vi "LinxI2cOpen.vi"(8 "Error In":errorcluster, 10 "I2C Channel":u8, 11 "LINX Resource":T1) -> (0 "Error Out":errorcluster, 3 "LINX Resource":T1)   [LabVIEW 2020, in "LMH-LINX.lvlib" / "Local IO.lvlib"]
uses:
  Local IO.lvlib
  Type Defs/LINX Ref.ctl
  Type Defs/Platform.ctl
  Type Defs/Interface.ctl
  Device/Type Defs/LINX Device Config.ctl
  Device/Type Defs/TCP Config.ctl
  Device/Type Defs/Channels.ctl
  <vilib>/MakerHub/LINX/Resources/liblinxdevice.dll
  LMH-LINX.lvlib
  Device/Device.lvlib
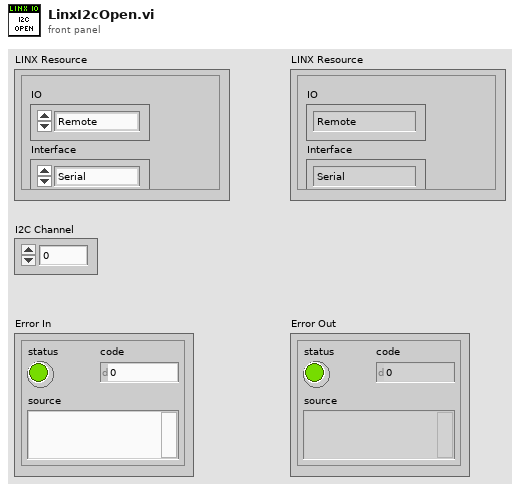
[diagram p1: front panel]
types:
  T1 = typedef "LMH-LINX.lvlib/LINX Ref.ctl" = cluster{"IO":T2, "Interface":T3, "LINX Device Config":T4}
  T2 = typedef "LMH-LINX.lvlib/Platform.ctl" = enum16{"Remote", "Local"}
  T3 = typedef "LMH-LINX.lvlib/Interface.ctl" = enum16{"Serial", "TCP"}
  T4 = typedef "LMH-LINX.lvlib/Device.lvlib/LINX Device Config.ctl" = cluster{"Interface":T3, "COM Port":refnum<visa-resource-name>, "TCP Configuration":T5, "Device Family":u8, "Device ID":u8, "Device Name":string, "TCP Ref":refnum<k5>, "Channels":T6}
  T5 = typedef "LMH-LINX.lvlib/Device.lvlib/TCP Config.ctl" = cluster{"IP Address":string, "Port":u16}
  T6 = typedef "LMH-LINX.lvlib/Channels.ctl" = cluster{"DI":u8[], "DO":u8[], "AI":u8[], "AO":u8[], "PWM":u8[], "QE":u8[], "UART":u8[], "I2C 2":u8[], "SPI":u8[], "CAN":u8[], "Servo":u8[], "AI Ref (V)":dbl, "AI Resolution (Bits)":u8, "AO Ref (V)":dbl, "AO Resolution (Bits)":u8}
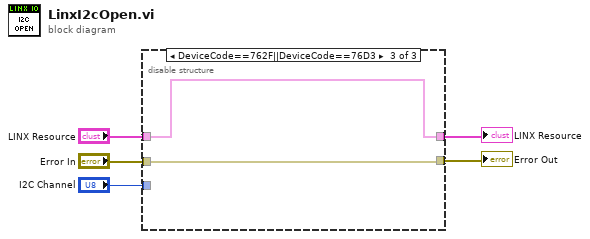
[diagram p0: block diagram]
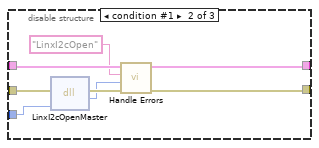
[diagram p3: hidden frame]
diagram:
  n1 = disable-structure shown="DeviceCode==762F||DeviceCode==76D3" {
    disable-tunnel: "LINX Resource" -> [w7 w14 w17]
    disable-tunnel: "Error In" -> [w6 w15 w16]
    disable-tunnel: [w6 w12 w16] -> w3
    disable-tunnel: [w7 w13 w17] -> w2
    disable-tunnel: "I2C Channel" -> [_ w8 _]
    frame condition #0 (active) {
    }
    frame condition #1 {
      n2 = dll-call lib="C:/Program Files (x86)/National Instruments/LabVIEW 2020/vi.lib/MakerHub/LINX/Resources/liblinxdevice.*" fn="LinxI2cOpenMaster"(error in=w15, "channel"=w8) -> (error out=w11:errorcluster, "LinxStatus"=w10:i32)  [unwired: 3 in, 1 out]
      n3 = call <vilib>:"Handle Errors.vi"("Error In"=w11, "LinxStatus"=w10, "Function Name"="LinxI2cOpen", "LINX Resource"=w14) -> ("Error Out"=w12:errorcluster, "LINX Resource"=w13:T1)  [unwired: 6 in]
    }
    frame condition #2 {
    }
  }
  "Error Out" <- w3
  "LINX Resource" <- w2
